vi "destroy.vi"(8 "error in (no error)":errorcluster, 11 "system in":refnum<class "system.lvclass">) -> (0 "error out":errorcluster)   [LabVIEW 2021, in "system.lvclass"]
uses:
  system.lvclass
  system.lvclass/system.ctl
  system.threading/system.threading.lvclass
  system.logging/system.logging.lvclass
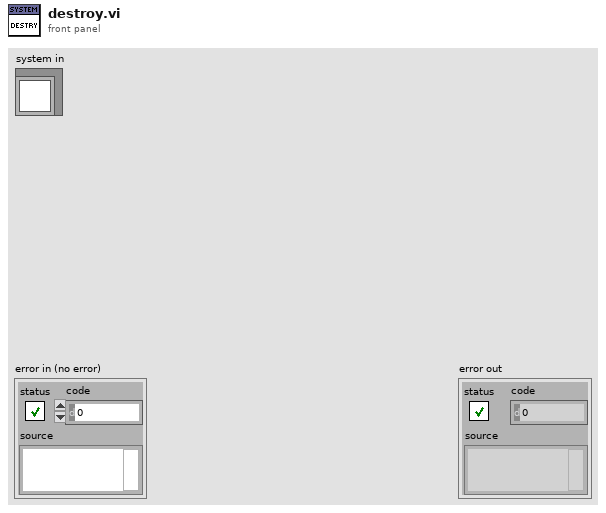
[diagram p1: front panel]
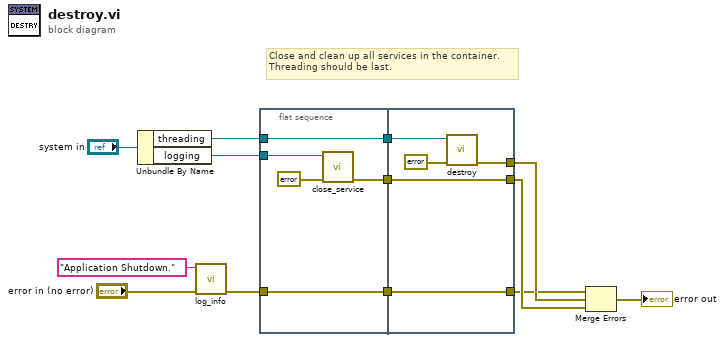
[diagram p0: block diagram]
diagram:
  # "Close and clean up all services in the container.\nThreading should be last."
  n1 = Unbundle By Name("system in") -> ("threading"=w10:refnum<class "system.threading.lvclass">, "logging"=w11:refnum<class "system.logging.lvclass">)
  n2 = call "log_info.vi"("error in (no error)"="error in (no error)", "message"="Application Shutdown.") -> ("error out"=w4:errorcluster)  [unwired: 9 in]
  n3 = flat-sequence {
    tunnel: w11 -> [w14]
    tunnel: w10 -> [w18]
    tunnel: [w18] -> w9
    tunnel: [w15] -> w8
    tunnel: w4 -> [w17]
    tunnel: [w17] -> w2
    tunnel: w9 -> [w22]
    tunnel: [w21] -> w7
    tunnel: w8 -> [w21]
    tunnel: [w20] -> w6
    tunnel: w2 -> [w19]
    tunnel: [w19] -> w1
    frame #0 {
      n4 = call "close_service.vi"("error in (no error)"=errorcluster {"status"=FALSE, "code"=0, "source"=""}, "system.logging (in)"=w14) -> ("error out"=w15:errorcluster)  [unwired: 8 in, 1 out]
    }
    frame #1 {
      n5 = call "destroy.vi"("error in (no error)"=errorcluster {"status"=FALSE, "code"=0, "source"=""} ("error constant"), "system.threading in"=w22) -> ("error out"=w20:errorcluster)  [unwired: 9 in]
    }
  }
  n6 = Merge Errors(w1, w6, w7) -> (→"error out":errorcluster)
